vi "Scale Output ADXL345.vi"(9 "Byte1":u8, 11 "Byte0":u8) -> (3 "G's":dbl)   [LabVIEW 2014]
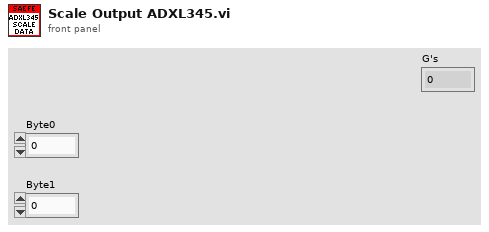
[diagram p1: front panel]
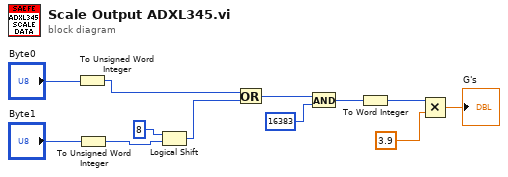
[diagram p0: block diagram]
diagram:
  n1 = To Unsigned Word Integer(number="Byte0") -> (unsigned 16bit integer=w8:u16)
  n2 = To Unsigned Word Integer(number="Byte1") -> (unsigned 16bit integer=w10:u16)
  n3 = Logical Shift(y=i16 8, x=w10) -> (x << y=w7:u16)
  n4 = Or(x=w8, y=w7) -> (x .or. y?=w6:u16)
  n5 = And(x=w6, y=u16 16383) -> (x .and. y?=w4:u16)
  n6 = To Word Integer(number=w4) -> (16bit integer=w3:i16)
  n7 = Multiply(x=w3, y=3.9) -> (x*y=→"G's":dbl)
